vi "MotorFun.vi"() -> ()   [LabVIEW 2019]
uses:
  <userlib>/MicroPython/VIs/uPythonX/uPythonX.xctl
panel:
  in  "uPythonX":T1(xcontrol)={"Port"="ASRL118::INSTR", "All Code"="import hub,utime\n\nhub.port.A.motor.get()\n\nhub.port.A.motor.run_for_degrees(90, speed = 50)\np.run_for_time(200,40,-40)\n\n\np = hub.port.A.motor.pair(hub.port.B.motor)\nl=hub.port.E.motor\nr=hub.port.F.motor\n\nl.mode(3)\nl.get()\nr.mode(3)\nr.get()\n\nl.run_to_position(-102,20)\nl.run_for_degrees(90, speed = 50)\n\n# it seems that run_degrees is a relative measure, \n#run position is also relative to where you are  but get is absolute\n\n# start by rotating both to zero and then plugging them in\n   \nl=hub.port.A.motor\nr=hub.port.B.motor\nl.mode(3)\nr.mode(3)\nl.run_to_position(-90,50,stop = l.STOP_HOLD)\nr.run_to_position(90,50,stop = l.STOP_HOLD)\nwhile 1:\n    # hub.sound.beep()\n    lstart = -90\n    rstart=90\n     for i in range(9):\n          l.run_to_position(lstart+i*10,20,stop = l.STOP_HOLD)\n          r.run_to_position(rstart-i*10,20,stop = l.STOP_HOLD)\n          utime.sleep(1)\n          pos = l.get()[0]\n          print ('%d:  %d -> %d' % (lstart+i*10-pos,lstart+i*10,pos))\n          pos = r.get()[0]\n          print ('%d:  %d -> %d' % (rstart-i*10-pos,rstart-i*10,pos))\n\n\np = hub.port.A.motor.pair(hub.port.B.motor)\nhip = hub.port.C.motor.pair(hub.port.D.motor)\n\np.run_to_position(-90,90,20,stop=2)\nhip.run_to_position(20,-20,20,stop=2)\n\np.run_to_position(-70,70,20,stop=2)\nhip.run_to_position(30,-30,20,stop=2)\n\np.run_to_position(-100,100,20,stop=2)\nhip.run_to_position(-50,50,20,stop=2)\n\np.run_to_position(-105,105,20,stop=2)\nhip.run_to_position(-60,60,20,stop=2)\n\np.run_to_position(-90,90,20,stop=2)\nhip.run_to_position(-0,0,20,stop=2)\n\n\nwhile 1:\n    # hub.sound.beep()\n    lstart = -90\n    rstart=90\n     for i in range(9):\n          p.run_to_position(lstart+i*10,rstart-i*10,20,stop=2)\n          utime.sleep(1)\n          pos = l.get()[0]\n          print ('%d:  %d -> %d' % (lstart+i*10-pos,lstart+i*10,pos))\n          pos = r.get()[0]\n          print ('%d:  %d -> %d' % (rstart-i*10-pos,rstart-i*10,pos))\nq``"}
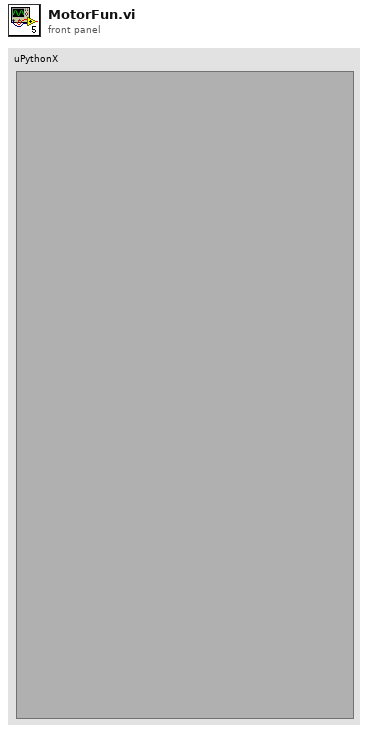
[diagram p1: front panel]
types:
  T1 = cluster{"Port":refnum<visa-resource-name>, "All Code":string}
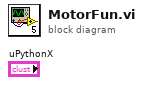
[diagram p0: block diagram]
diagram:
